vi "MCLB.vi"(11 "Error_In":errorcluster) -> (4 "Multicolumn_Listbox":i32[](listbox), 15 "Errror_Out":errorcluster)   [LabVIEW 2021]
uses:
  <vilib>/Utility/miscctls.llb/LVPositionTypeDef.ctl
  Controls/Names_Box.ctl
panel:
  in  "Names_Box":T1
  # "Solins List and Track"
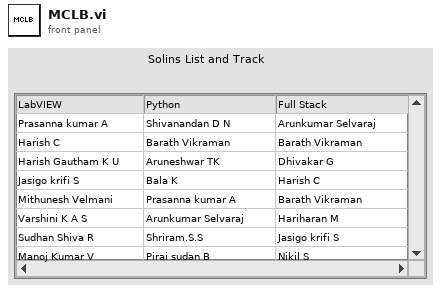
[diagram p1: front panel]
types:
  T1 = typedef "Names_Box.ctl" = string
  T2 = typedef "LVPositionTypeDef.ctl" = cluster{"Left":i32, "Top":i32}
  T3 = typedef "LVPoint32TypeDef.ctl" = cluster{"Horizontal":i32, "Vertical":i32}
  T4 = typedef "LVRowAndColumnTypeDef.ctl" = cluster{"Row":i32, "Column":i32}
  T5 = enum16{"Left Button", "Center Button", "Right Button", "Window Close"}
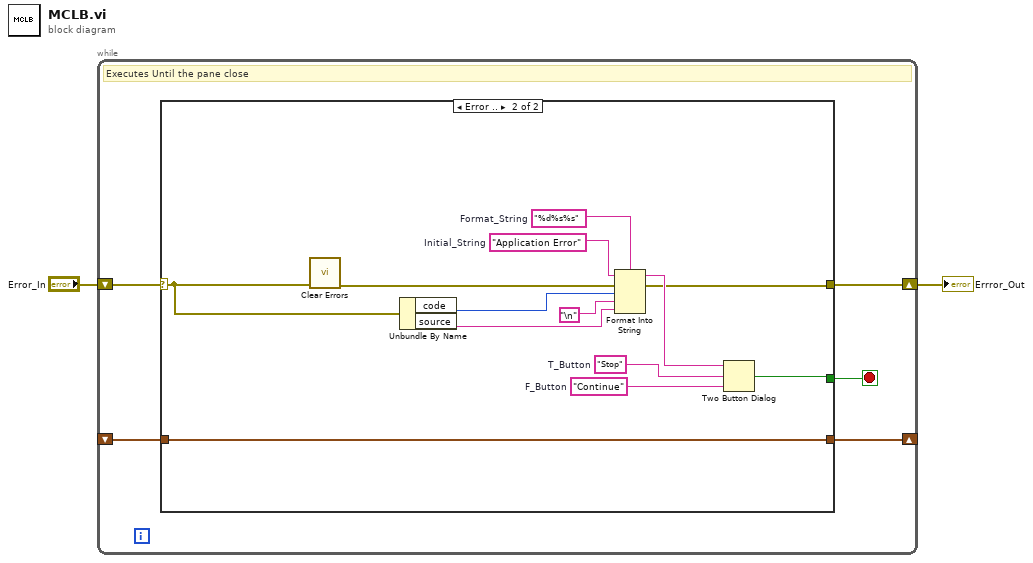
[diagram p0: block diagram]
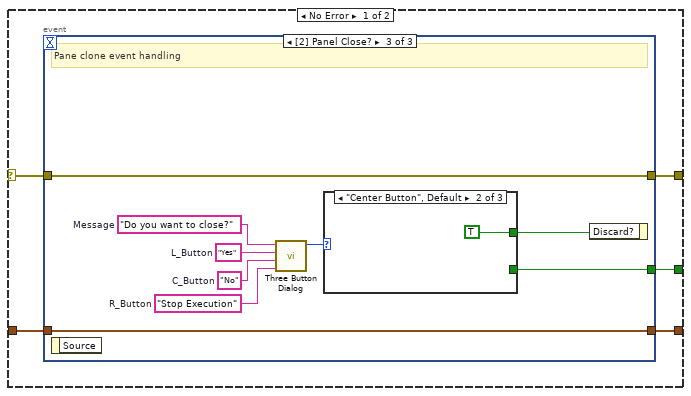
[diagram p2: hidden frame]
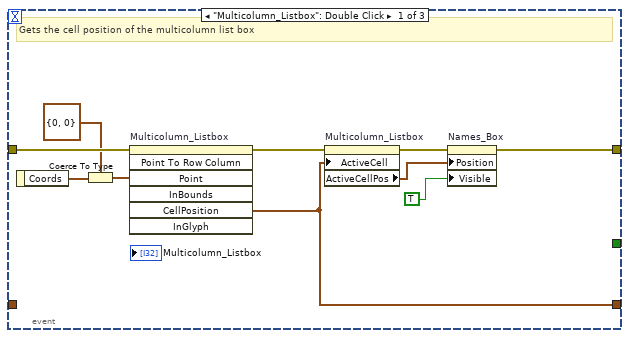
[diagram p3: hidden frame]
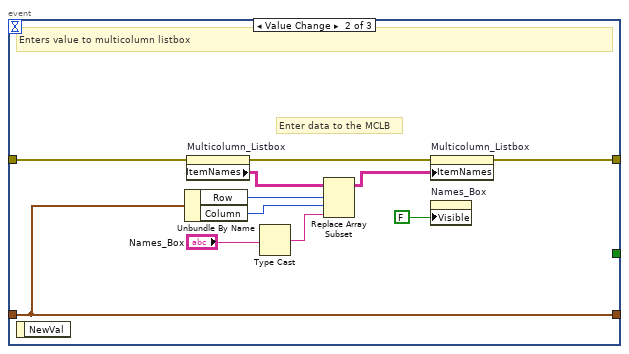
[diagram p4: hidden frame]
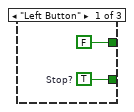
[diagram p5: hidden frame]
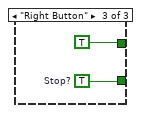
[diagram p6: hidden frame]
diagram:
  n1 = while {
    shift-right: [w6] -> _
    shift-left: _ -> [w7]
    shift-right: [w3] -> w1
    shift-left: "Error_In" -> [w4]
    stop <- w5 stop-if-true
    # "Executes Until the pane close"
    n2 = case shown="Error .." w4 {
      selector: w4 -> [w9 w51]
      tunnel: w7 -> [w12 w49]
      tunnel: [w11 w49] -> w6
      tunnel: [w10 w48] -> w5
      tunnel: [w8 w50] -> w3
      frame No Error {
        n3 = event shown="[2] Panel Close?" {
          selector: _ -> [_ _ _]
          dyn-events: _ -> [_ _ _]
          timeout: _ -> [_ _ _]
          tunnel: w12 -> [_ w29 w42]
          tunnel: [w21 w29 w42] -> w11
          tunnel: [_ _ w35] -> w10
          tunnel: w9 -> [w19 w27 w34]
          tunnel: [w16 w25 w34] -> w8
          event "Multicolumn_Listbox": Double Click {
            # "Gets the cell position of the multicolumn list box"
            n4 = event-data() -> ("Coords"=w15:T3)  [unwired: 1 in]
            n5 = Coerce To Type(0:w15, 1:T2 {"Left"=0, "Top"=0} ("Point")) -> (2:w13:T2)
            n6 = invoke on="Multicolumn_Listbox" class="MCListbox (strict)" method="Point To Row Column"(error in=w19, "Point"=w13) -> (error out=w18:errorcluster, "CellPosition"=w21:T4)  [unwired: 5 in, 5 out]
            n7 = property on="Multicolumn_Listbox" class="MCListbox (strict)"(error in=w18, "ActiveCell"=w21) -> (error out=w17:errorcluster, "ActiveCellPos"=w22:T2)  [unwired: 1 in, 1 out]
            n8 = property on="Names_Box" class="CmbBox (strict)"(error in=w17, "Position"=w22, "Visible"=TRUE) -> (error out=w16:errorcluster)  [unwired: 1 in, 1 out]
          }
          event Value Change {
            # "Enter data to the MCLB"
            # "Enters value to multicolumn listbox"
            n9 = event-data() -> ()  [unwired: 1 in, 1 out]
            n10 = Unbundle By Name(w29) -> ("Row"=w30:i32, "Column"=w31:i32)
            n11 = property on="Multicolumn_Listbox" class="MCListbox (strict)"(error in=w27) -> (error out=w26:errorcluster, "ItemNames"=w28:string[][])  [unwired: 1 in, 1 out]
            n12 = Type Cast(x="Names_Box") -> (*(type *) &x=w23:string)  [unwired: 1 in]
            n13 = Replace Array Subset(array=w28, new element=w23, index (row)=w30, index (col)=w31) -> (w32:string[][])
            n14 = property on="Multicolumn_Listbox" class="MCListbox (strict)"(error in=w26, "ItemNames"=w32) -> (error out=w25:errorcluster)  [unwired: 1 in, 1 out]
            n15 = property on="Names_Box" class="CmbBox (strict)"("Visible"=FALSE) -> ()  [unwired: 2 in, 2 out]
          }
          event Panel Close? {
            w38 = "Stop Execution"  # R_Button
            w39 = "No"  # C_Button
            w40 = "Yes"  # L_Button
            w41 = "Do you want to close?"  # Message
            # "Pane clone event handling"
            n16 = event-data() -> ()  [unwired: 1 in, 1 out]
            n17 = call <vilib>:"Three Button Dialog.vi"("Right Button Text (\"Cancel\")"=w38, "Center Button Text (\"No\")"=w39, "Left Button Text (\"Yes\")"=w40, "message"=w41) -> ("Which Button?"=w37:T5)  [unwired: 7 in]
            n18 = case shown="\"Center Button\", Default" w37 {
              tunnel: [FALSE TRUE TRUE] -> w36
              tunnel: [w43 _ w47] -> w35
              frame "Left Button" {
                w43 = TRUE  # Stop?
              }
              frame "Center Button", Default {
              }
              frame "Right Button" {
                w47 = TRUE  # Stop?
              }
            }
            n19 = event-data("Discard?"=w36) -> ()  [unwired: 1 in, 1 out]
          }
        }
      }
      frame Error {
        w53 = "%d%s%s"  # Format_String
        w54 = "Application Error"  # Initial_String
        w55 = "Stop"  # T_Button
        w56 = "Continue"  # F_Button
        n20 = call <vilib>:"Clear Errors.vi"("error in (no error)"=w51) -> ("error out"=w58:errorcluster)  [unwired: 5 in, 1 out]
        n21 = Unbundle By Name(w51) -> ("code"=w60:i32, "source"=w59:string)
        n22 = Format Into String(format string=w53, initial string=w54, error in=w58, w60, "\n", w59) -> (resulting string=w57:string, error out=w50:errorcluster)
        n23 = Two Button Dialog(message=w57, 1:w56, 2:w55) -> (T button?=w48:bool)
      }
    }
  }
  "Errror_Out" <- w1
